vi "Write display name.vi"(8 "error in":errorcluster, 10 "display name":string, 11 "module editor node in":refnum<class "module editor node.lvclass">) -> (0 "error out":errorcluster, 3 "module editor node out":refnum<class "module editor node.lvclass">)   [LabVIEW 2013, in "PL Framework Configuration Tool.lvlib" / "module editor node.lvclass"]
uses:
  module editor node.lvclass
  <vilib>/NI/Configuration Framework/serializable configuration/NISE_CEF_serializable configuration.lvclass
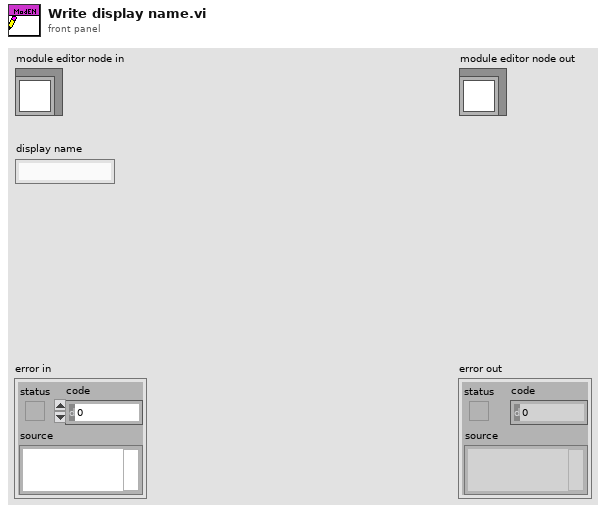
[diagram p1: front panel]
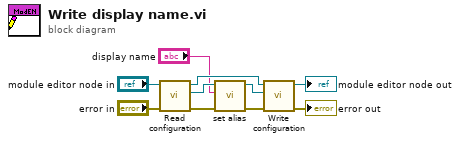
[diagram p0: block diagram]
diagram:
  n1 = call-dynamic "Read configuration.vi"("error in"="error in", "NISE_CEF_serializable node in"="module editor node in") -> ("error out"=w3:errorcluster, "configuration"=w4:refnum<class "NISE_CEF_serializable configuration.lvclass">, "NISE_CEF_serializable node out"=w6:refnum<class "module editor node.lvclass">)  [unwired: 7 in]
  n2 = call <vilib>:"set alias.vi"("error in"=w3, "alias"="display name", "configuration in"=w4) -> ("error out"=w1:errorcluster, "configuration out"=w5:refnum<class "NISE_CEF_serializable configuration.lvclass">)  [unwired: 7 in]
  n3 = call-dynamic "Write configuration.vi"("error in"=w1, "configuration"=w5, "NISE_CEF_serializable node in"=w6) -> ("error out"=→"error out":errorcluster, "NISE_CEF_serializable node out"=→"module editor node out":refnum<class "module editor node.lvclass">)  [unwired: 7 in]
